vi "ArmCurls.vi"(9 "Actual Shoulder Angle (deg)":dbl, 10 "Elbow Speed":dbl, 11 "shoulder speed (deg/s)":dbl) -> ()   [LabVIEW 2018]
uses:
  <vilib>/Rock Robotics/Network Tables/NT Write Number.vi
panel:
  out "Elbow Speed 2":dbl
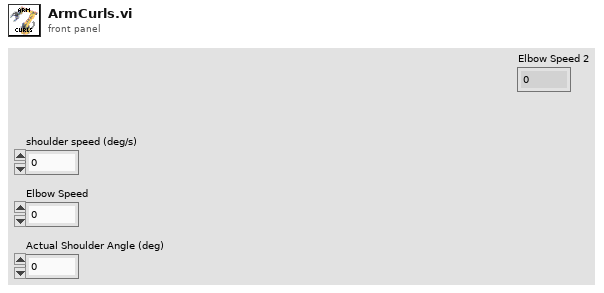
[diagram p1: front panel]
types:
  T1 = typedef "WPI_MotorControlDeviceRef.ctl" = cluster{"DeviceStatus":errorcluster, "Type":T2, "PWM":cluster{"PWM Channel":T3, "DeadBand":T4}, "CAN":cluster{"Device Number":u8, "SetOutput VI Ref":variant, "GetOutput VI Ref":variant, "Enable VI Ref":variant, "Disable VI Ref":variant, "Data":variant}, "Invert":bool, "DIO PWM":cluster{"PWM \"Enable\" Channel":T3, "DIOChannel":T5, "PWM Rate":dbl}}
  T2 = typedef "WPI_MotorControlType.ctl" = enum16{"PWM", "CAN", "DIO PWM"}
  T3 = typedef "FPGA_DIOPWMChannel.ctl" = enum8{"PWM 0", "PWM 1", "PWM 2", "PWM 3", "PWM 4", "PWM 5", "PWM 6", "PWM 7", "PWM 8", "PWM 9", "PWM MXP 0", "PWM MXP 1", "PWM MXP 2", "PWM MXP 3", "PWM MXP 4", "PWM MXP 5", "PWM MXP 6", "PWM MXP 7", "PWM MXP 8", "PWM MXP 9", "Invalid"}
  T4 = typedef "WPI_PWMDeadband.ctl" = cluster{"Name":string, "maxPositivePwm":i32, "minPositivePwm":i32, "centerPwm":i32, "maxNegativePwm":i32, "minNegativePwm":i32, "angularRange":u16}
  T5 = typedef "FPGA_DIOChannel.ctl" = enum8{"DIO 0", "DIO 1", "DIO 2", "DIO 3", "DIO 4", "DIO 5", "DIO 6", "DIO 7", "DIO 8", "DIO 9", "DIO MXP 0", "DIO MXP 1", "DIO MXP 2", "DIO MXP 3", "DIO MXP 4", "DIO MXP 5", "DIO MXP 6", "DIO MXP 7", "DIO MXP 8", "DIO MXP 9", "DIO MXP 10", "DIO MXP 11", "DIO MXP 12", "DIO MXP 13", "DIO MXP 14", "DIO MXP 15", "SPI Port CS1", "SPI Port CS2", "SPI Port CS3", "SPI Port MISO", "SPI Port MOSI", "Invalid"}
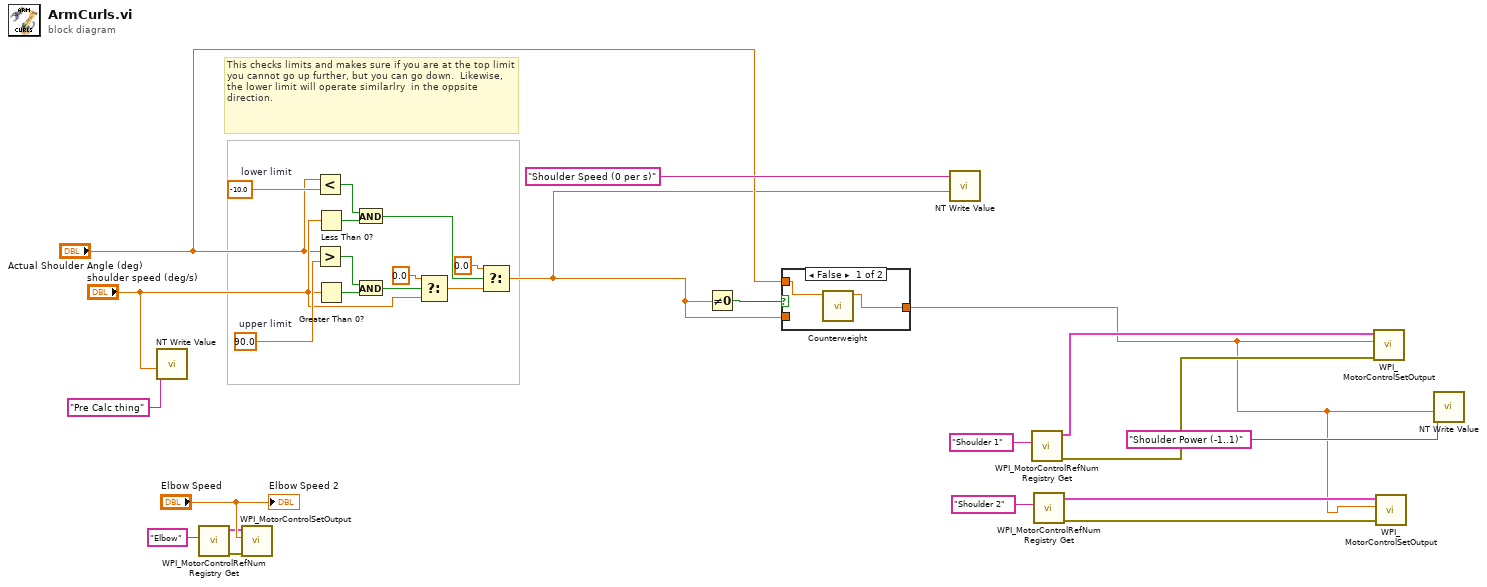
[diagram p0: block diagram]
diagram:
  w15 = -10.0  # lower limit
  w24 = 90.0  # upper limit
  # "This checks limits and makes sure if you are at the top limit you cannot go up further, but you can go down.  Likewise, the lower limit will operate similarlry  in the oppsite direction."
  n1 = call-poly <vilib>:"NT Write Value.vi"("Numeric"="shoulder speed (deg/s)", "Name"="Pre Calc thing") -> ()  [unwired: 9 in, 1 out]
  n2 = call <vilib>:"WPI_MotorControlRefNum Registry Get.vi"("refnum name"="Elbow") -> ("error out"=w12:errorcluster, "MotorControlDevRef"=w13:T1)  [unwired: 9 in]
  n3 = call <vilib>:"WPI_MotorControlSetOutput.vi"("error in (no error)"=w12, "Output"="Elbow Speed", "MotorControlDevRef"=w13) -> ()  [unwired: 6 in, 3 out]
  n4 = Less?(x="Actual Shoulder Angle (deg)", y=w15) -> (x < y?=w17:bool)
  n5 = Greater?(x="Actual Shoulder Angle (deg)", y=w24) -> (0:w22:bool)
  n6 = Less Than 0?(x="shoulder speed (deg/s)") -> (x < 0?=w16:bool)
  n7 = Greater Than 0?(x="shoulder speed (deg/s)") -> (x > 0?=w23:bool)
  n8 = And(x=w17, y=w16) -> (x .and. y?=w18:bool)
  n9 = And(x=w22, y=w23) -> (x .and. y?=w21:bool)
  n10 = Select(t=0.0 ("f"), s=w21, f="shoulder speed (deg/s)") -> (s? t:f=w14:dbl)
  n11 = Select(t=0.0 ("f"), s=w18, f=w14) -> (s? t:f=w2:dbl)
  n12 = Not Equal To 0?(x=w2) -> (x != 0?=w3:bool)
  n13 = case shown="False" w3 {
    tunnel: "Actual Shoulder Angle (deg)" -> [w31 _]
    tunnel: [w30 w32] -> w1
    tunnel: w2 -> [_ w32]
    frame False {
      n14 = call "Counterweight.vi"("Current Angle"=w31) -> ("Current Counter Weight Power"=w30:dbl)  [unwired: 10 in]
    }
    frame True {
    }
  }
  n15 = call-poly <vilib>:"NT Write Value.vi"("Numeric"=w2, "Name"="Shoulder Speed (0 per s)") -> ()  [unwired: 9 in, 1 out]
  n16 = call <vilib>:"WPI_MotorControlRefNum Registry Get.vi"("refnum name"="Shoulder 1") -> ("error out"=w26:errorcluster, "MotorControlDevRef"=w27:T1)  [unwired: 9 in]
  n17 = call <vilib>:"WPI_MotorControlRefNum Registry Get.vi"("refnum name"="Shoulder 2") -> ("error out"=w10:errorcluster, "MotorControlDevRef"=w9:T1)  [unwired: 9 in]
  n18 = call <vilib>:"WPI_MotorControlSetOutput.vi"("error in (no error)"=w26, "Output"=w1, "MotorControlDevRef"=w27) -> ()  [unwired: 6 in, 3 out]
  n19 = call <vilib>:"WPI_MotorControlSetOutput.vi"("error in (no error)"=w10, "Output"=w1, "MotorControlDevRef"=w9) -> ()  [unwired: 6 in, 3 out]
  n20 = call-poly <vilib>:"NT Write Value.vi"("Numeric"=w1, "Name"="Shoulder Power (-1..1)") -> ()  [unwired: 9 in, 1 out]
  "Elbow Speed 2" <- "Elbow Speed"
